vi "Fdx Create Tx VL.vi"(8 "error in (no error)":errorcluster, 10 "VL Config":T1={"VlId"=1, "NumOfSubVl"=1, "rate ms [Bag]"=128, "domainID"=1, "sideID"=1, "locationID"=1, "interfaceID"=1, "NetSelect"=3, "Skew"=0, "MaxFrameLength"=1000, "FrameBufferSize"=0} {"NetSelect" items=["FDX_TX_FRAME_DLY_A"=0, "FDX_TX_FRAME_DLY_B"=1, "FDX_TX_FRAME_BOTH "=3, "FDX_TX_FRAME_ONLY_A"=4, "FDX_TX_FRAME_ONLY_B "=5]; "interfaceID" format="%.0b"}, 11 "InstrumentHandle in":u32) -> (0 "error out":errorcluster, 1 "VlId":u16, 3 "InstrumentHandle out":u32)   [LabVIEW 2020, in "AIM664LV.lvlib"]
doc: "This function is used to setup a Virtual Link to transmit data. This is only a description of the Virtual Link specific parameters, which must be known by the system for transmitting. This function can be used only when the transmitter is not running."
uses:
  AIM664LV.lvlib
  _controls/comm_config_vl_tx.ctl
  helpers/EthFrameManagement/controls/mac_src_info_afdx.ctl
  helpers/EthFrameManagement/EthFrameManagement.lvlib
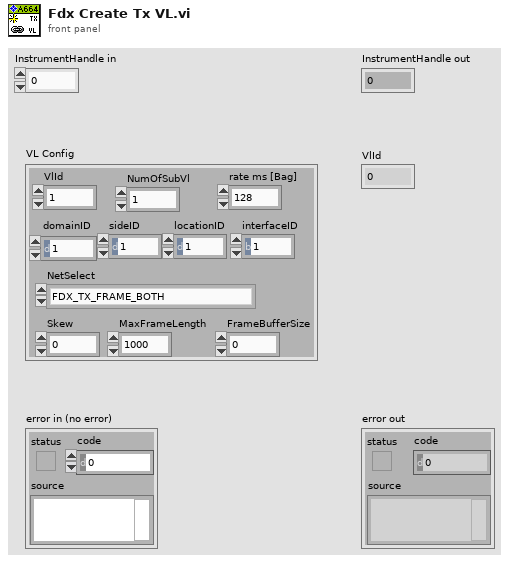
[diagram p1: front panel]
types:
  T1 = typedef "AIM664LV.lvlib/comm_config_vl_tx.ctl" = cluster{"VlId":u16, "NumOfSubVl":u16, "rate ms [Bag]":u32, "domainID":u8, "sideID":u8, "locationID":u8, "interfaceID":u8, "NetSelect":u32, "Skew":u32, "MaxFrameLength":u32, "FrameBufferSize":u32}
  T2 = cluster{"VlId":u32, "SubVls":u32, "Bag":u32, "NetSelect":u32, "MaxFrameLength":u32, "FrameBufferSize":u32, "MACSourceLSLW":u32, "MACSourceMSLW":u32, "Skew":u32}
  T3 = typedef "EthFrameManagement.lvlib/mac_src_info_afdx.ctl" = cluster{"domainID":u8, "sideID":u8, "locationID":u8, "interfaceID":u8}
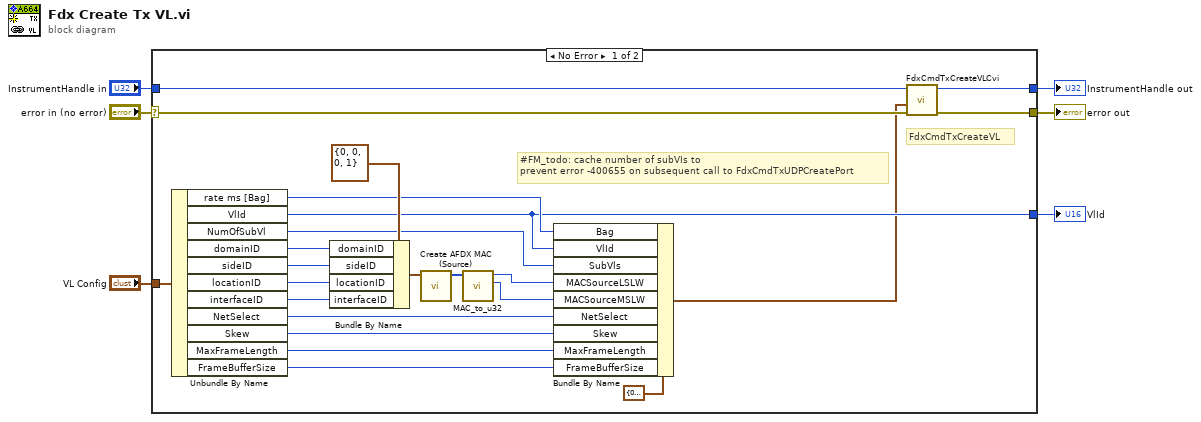
[diagram p0: block diagram]
diagram:
  n1 = case shown="No Error" "error in (no error)" {
    selector: "error in (no error)" -> [w26 w31]
    tunnel: [w11 w31] -> w5
    tunnel: [w7 w30] -> w3
    tunnel: "InstrumentHandle in" -> [w12 w30]
    tunnel: "VL Config" -> [w29 _]
    tunnel: [w10 _] -> w1
    frame No Error {
      # "FdxCmdTxCreateVL"
      # "#FM_todo: cache number of subVIs to\nprevent error -400655 on subsequent call to FdxCmdTxUDPCreatePort"
      n2 = Unbundle By Name(w29) -> ("rate ms [Bag]"=w24:u32, "VlId"=w10:u16, "NumOfSubVl"=w23:u16, "domainID"=w20:u8, "sideID"=w19:u8, "locationID"=w18:u8, "interfaceID"=w17:u8, "NetSelect"=w16:u32, "Skew"=w15:u32, "MaxFrameLength"=w14:u32, "FrameBufferSize"=w13:u32)
      n3 = Bundle By Name(cluster=T3 {"domainID"=0, "sideID"=0, "locationID"=0, "interfaceID"=1} ("Source Info"), "domainID"=w20, "sideID"=w19, "locationID"=w18, "interfaceID"=w17) -> (w8:T3)
      n4 = call "Create AFDX MAC (Source).vi"("Source Info"=w8) -> ("MAC-src"=w28:u8[])  [unwired: 10 in]
      n5 = call "MAC_to_u32.vi"("MAC (aa:bb:cc:dd:ee:ff)"=w28) -> ("MSLW"=w21:u32, "LSLW"=w22:u32)  [unwired: 9 in]
      n6 = Bundle By Name(cluster=T2 {"VlId"=0, "SubVls"=0, "Bag"=0, "NetSelect"=0, "MaxFrameLength"=0, "FrameBufferSize"=0, "MACSourceLSLW"=0, "MACSourceMSLW"=0, "Skew"=0} ("Input Cluster"), "Bag"=w24, "VlId"=w10, "SubVls"=w23, "MACSourceLSLW"=w22, "MACSourceMSLW"=w21, "NetSelect"=w16, "Skew"=w15, "MaxFrameLength"=w14, "FrameBufferSize"=w13) -> (w9:T2)
      n7 = call "FdxCmdTxCreateVLCvi.vi"("error in"=w26, "Input Cluster"=w9, "InstrumentHandle_port in"=w12) -> ("error out"=w11:errorcluster, "InstrumentHandle_port out"=w7:u32)  [unwired: 7 in]
    }
    frame Error {
    }
  }
  "error out" <- w5
  "InstrumentHandle out" <- w3
  "VlId" <- w1
